vi "ToString.vi"(1 "WebSocket":refnum<class "WebSocket.lvclass">) -> (0 "String":string)   [LabVIEW 2023, in "WebSocket.lvclass"]
uses:
  WebSocket.lvclass
  WebSocket.lvclass/WebSocket.ctl
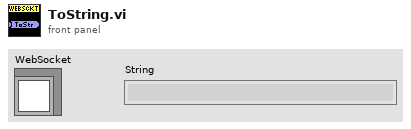
[diagram p1: front panel]
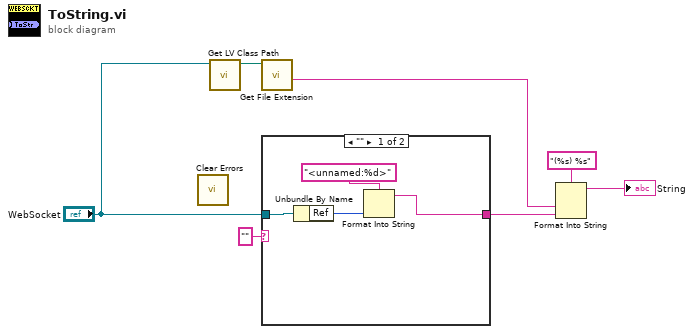
[diagram p0: block diagram]
diagram:
  n1 = call <vilib>:"Clear Errors.vi"() -> ()  [unwired: 6 in, 2 out]
  n2 = call <vilib>:"Get LV Class Path.vi"("object"="WebSocket") -> ("class path"=w7:path)  [unwired: 9 in, 1 out]
  n3 = call <vilib>:"Get File Extension.vi"("file"=w7) -> ("filename without extension"=w3:string)  [unwired: 6 in, 4 out]
  n4 = case shown="\"\"" "" {
    selector: "" -> [_ w12]
    tunnel: "WebSocket" -> [w11 _]
    tunnel: [w9 w12] -> w6
    frame "" {
      n5 = Unbundle By Name(w11) -> ("Ref"=w10:u32)
      n6 = Format Into String(format string="<unnamed:%d>", w10) -> (resulting string=w9:string)  [unwired: 2 in, 1 out]
    }
    frame Default {
    }
  }
  n7 = Format Into String(format string="(%s) %s", w3, w6) -> (resulting string=→"String":string)  [unwired: 2 in, 1 out]
